vi "Read Publisher Instance.vi"(8 "error in":errorcluster, 11 "CIFCorePlugin in":refnum<class "CIFCorePlugin.lvclass">) -> (0 "error out":errorcluster, 2 "Publisher Instance":T1, 3 "CIFCorePlugin out":refnum<class "CIFCorePlugin.lvclass">)   [LabVIEW 2021, in "CIFCorePlugin.lvclass"]
uses:
  CIFCorePlugin.lvclass
  Common/Typedef/FIFO Publisher.ctl
  <vilib>/CIF Foundation/CIF Channels Core/ChannelCommon/typedef/New FIFO Instance Configuration.ctl
  CIFCorePlugin.lvclass/CIFCorePlugin.ctl
  <vilib>/CIF Foundation/CIF Channels Core/ChannelCommon/ChannelCommon.lvlib
  Common/CIFCoreCommon.lvlib
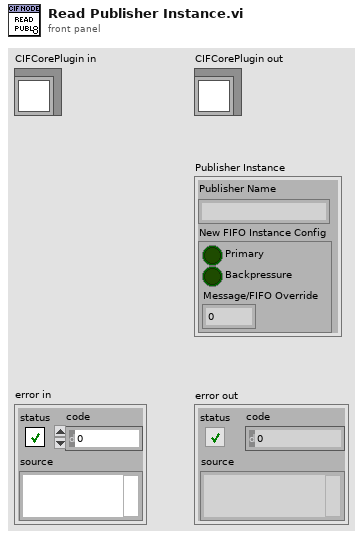
[diagram p1: front panel]
types:
  T1 = typedef "CIFCoreCommon.lvlib/FIFO Publisher.ctl" = cluster{"Publisher Name":string, "New FIFO Instance Config":T2}
  T2 = typedef "ChannelCommon.lvlib/New FIFO Instance Configuration.ctl" = cluster{"Primary":bool, "Backpressure":bool, "Message/FIFO Override":u32}
  T3 = typedef "CIFCorePlugin.lvclass/gRPC to Main DVR.ctl" = refnum<data-value>
  T4 = typedef "CIFCoreCommon.lvlib/gRPC to Main Data.ctl" = cluster{"Config Data":variant, "Connection":T5, "Force":T6, "Clock Conversion":T7, "Publisher Instance":T1}
  T5 = typedef "CIFCoreCommon.lvlib/Channel Connection Data.ctl" = cluster{"Publisher Name":string, "Subscriber Name":string, "Connection Data":u8[]}
  T6 = typedef "CIFCoreCommon.lvlib/Channel Force Data.ctl" = cluster{"Channel Name":string, "Force Data":u8[], "Force Active":bool}
  T7 = typedef "Time_CIF_U.lvlib/Clock Conversion Map.ctl" = map{u8, cluster{"Last Reset":i64, "Offset Pair":T8, "Slope":dbl, "1/Slope":dbl}}
  T8 = typedef "Time_CIF_U.lvlib/Timestamp Pair.ctl" = cluster{"System Time":i64, "External Time":i64}
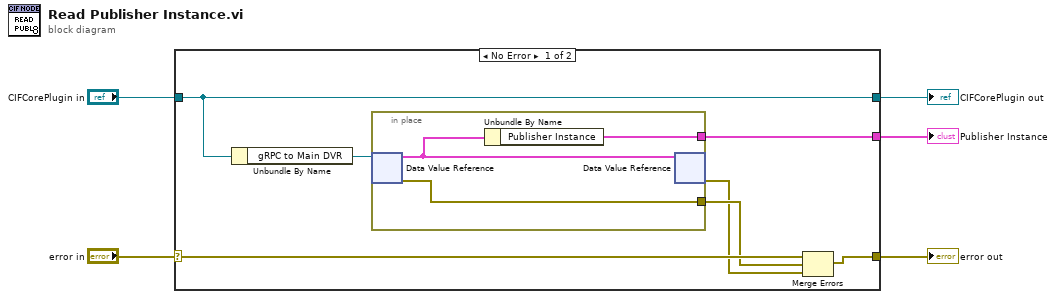
[diagram p0: block diagram]
diagram:
  n1 = case shown="No Error" "error in" {
    selector: "error in" -> [w10 w17]
    tunnel: [w6 w17] -> w4
    tunnel: "CIFCorePlugin in" -> [w12 w16]
    tunnel: [w12 w16] -> w2
    tunnel: [w9 _] -> w1
    frame No Error {
      n2 = Unbundle By Name(w12) -> ("gRPC to Main DVR"=w11:T3)
      n3 = in-place {
        in-place-border: [w14] -> w9
        in-place-border: [w13] -> w8
        n4 = in-place-dvr #1(w11) -> (w15:T4, w13:errorcluster)
        n5 = Unbundle By Name(w15) -> ("Publisher Instance"=w14:T1)
        n6 = in-place-dvr #1(w15) -> (w7:errorcluster)  [unwired: 1 out]
      }
      n7 = Merge Errors(w10, w8, w7) -> (w6:errorcluster)
    }
    frame Error {
    }
  }
  "Publisher Instance" <- w1
  "error out" <- w4
  "CIFCorePlugin out" <- w2
